vi "onVideoOptInfoUpd.vi"(8 "error in (no error)":errorcluster, 10 "VideoOptionsInfo":T1, 11 "CameraTestingUI in":refnum<class "CameraTestingUI.lvclass">) -> (0 "error out":errorcluster, 3 "CameraTestingUI out":refnum<class "CameraTestingUI.lvclass">)   [LabVIEW 2020, in "CameraTestingUI.lvlib" / "CameraTestingUI.lvclass"]
uses:
  CameraTestingUI.lvclass
  CameraTestingUI.lvclass/CameraTestingUI.ctl
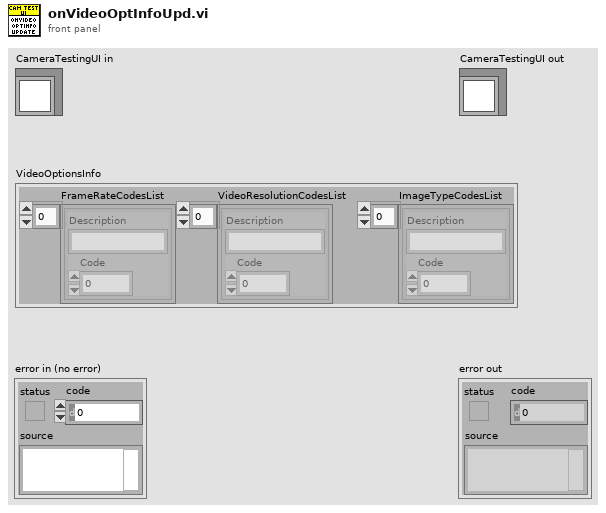
[diagram p1: front panel]
types:
  T1 = cluster{"FrameRateCodesList":cluster{"Description":string, "Code":u8}[], "VideoResolutionCodesList":cluster{"Description":string, "Code":u8}[], "ImageTypeCodesList":cluster{"Description":string, "Code":u8}[]}
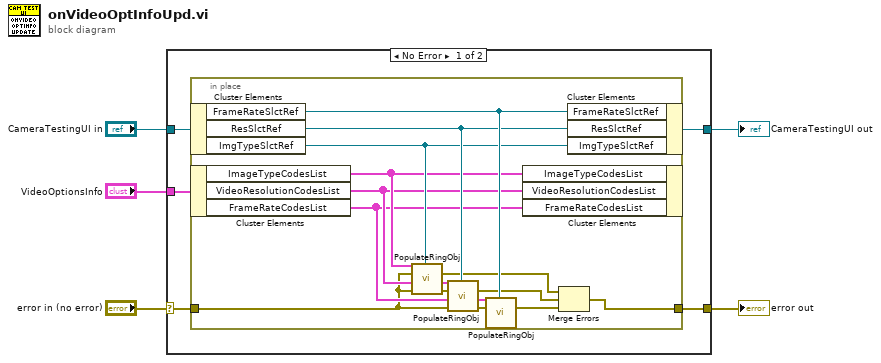
[diagram p0: block diagram]
diagram:
  n1 = case shown="No Error" "error in (no error)" {
    selector: "error in (no error)" -> [w8 w23]
    tunnel: [w6 w23] -> w4
    tunnel: [w7 w22] -> w2
    tunnel: "CameraTestingUI in" -> [w10 w22]
    tunnel: "VideoOptionsInfo" -> [w9 _]
    frame No Error {
      n2 = in-place {
        in-place-border: w8 -> [w15]
        in-place-border: [w11] -> w6
        n3 = in-place-cluster #1(w10) -> ("FrameRateSlctRef"=w21:refnum<vi>, "ResSlctRef"=w20:refnum<vi>, "ImgTypeSlctRef"=w19:refnum<vi>)
        n4 = in-place-cluster #2(w9) -> ("ImageTypeCodesList"=w18:cluster{"Description":string, "Code":u8}[], "VideoResolutionCodesList"=w17:cluster{"Description":string, "Code":u8}[], "FrameRateCodesList"=w16:cluster{"Description":string, "Code":u8}[])
        n5 = call "PopulateRingObj.vi"("Data []"=w18, "error in (no error)"=w15, "reference"=w19) -> ("error out"=w14:errorcluster)  [unwired: 24 in]
        n6 = call "PopulateRingObj.vi"("Data []"=w17, "error in (no error)"=w15, "reference"=w20) -> ("error out"=w13:errorcluster)  [unwired: 24 in]
        n7 = call "PopulateRingObj.vi"("Data []"=w16, "error in (no error)"=w15, "reference"=w21) -> ("error out"=w12:errorcluster)  [unwired: 24 in]
        n8 = in-place-cluster #2("ImageTypeCodesList"=w18, "VideoResolutionCodesList"=w17, "FrameRateCodesList"=w16) -> ()  [unwired: 1 out]
        n9 = Merge Errors(w14, w13, w12) -> (w11:errorcluster)
        n10 = in-place-cluster #1("FrameRateSlctRef"=w21, "ResSlctRef"=w20, "ImgTypeSlctRef"=w19) -> (w7:refnum<class "CameraTestingUI.lvclass">)
      }
    }
    frame Error {
    }
  }
  "error out" <- w4
  "CameraTestingUI out" <- w2
